vi "Controls State (array).vi"(8 "error in":errorcluster, 10 "Disabled":T1(ring), 11 "Controls Refnum":refnum<vi>[](array[refnum])) -> (0 "error out":errorcluster)   [LabVIEW 2020, in "Enum Queue State Machine.lvlib"]
uses:
  Enum Queue State Machine.lvlib
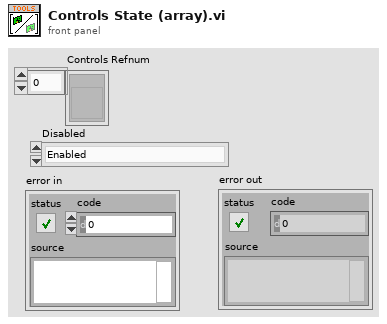
[diagram p1: front panel]
types:
  T1 = enum8{"Enabled", "Disabled", "Disabled and Grayed Out"}
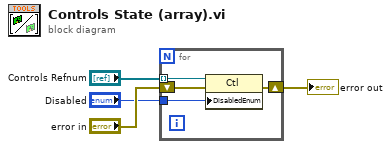
[diagram p0: block diagram]
diagram:
  n1 = for {
    tunnel: "Controls Refnum" -> [w8] mode=indexing
    tunnel: "Disabled" -> [w5]
    shift-right: [w6] -> w2
    shift-left: "error in" -> [w7]
    n2 = property class="Ctl"(reference=w8, error in=w7, "DisabledEnum"=w5) -> (error out=w6:errorcluster)  [unwired: 1 out]
  }
  "error out" <- w2
